vi "aggregator - i.vi"(5 "requested averaging interval":i32=1, 6 "first time":bool=TRUE, 7 "requested size":i32=1, 11 "number":cdb) -> (0 "interpolated average":cdb, 1 "mean array":cdb[](array[numeric]), 2 "interp array":cdb[](array[numeric]), 3 "Array":cdb[](array[numeric]), 4 "standard deviation":cdb[](array[numeric]))   [LabVIEW 2015]
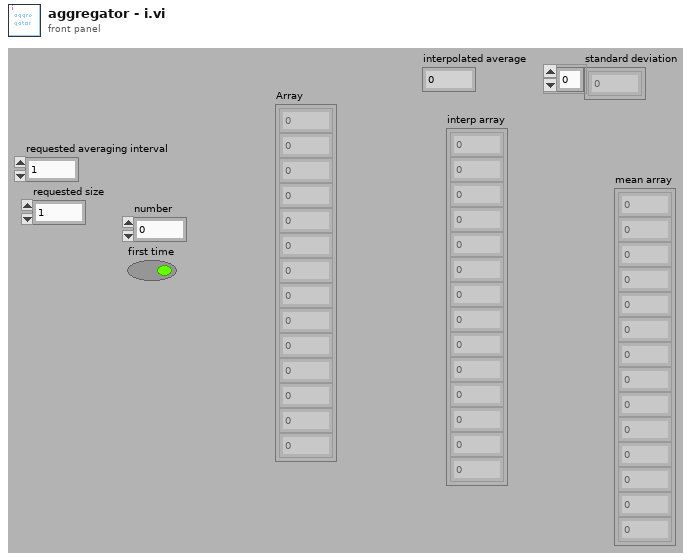
[diagram p1: front panel]
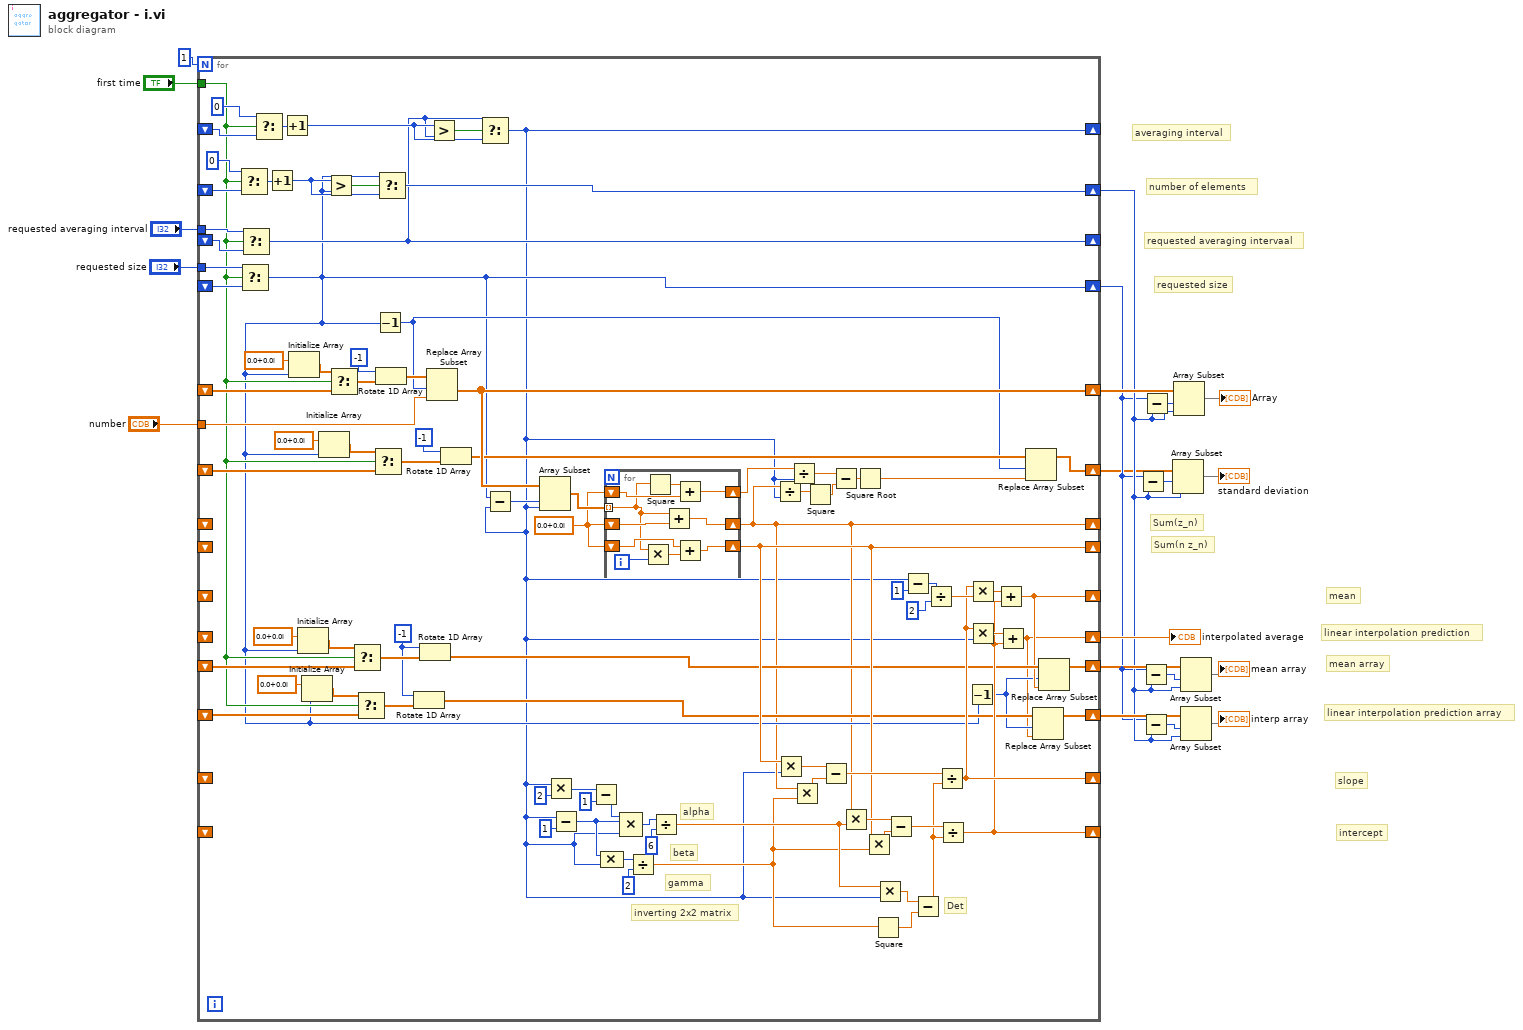
[diagram p0: block diagram]
diagram:
  # "averaging interval"
  # "requested averaging intervaal"
  # "linear interpolation prediction"
  # "mean"
  # "intercept"
  # "slope"
  # "linear interpolation prediction array"
  # "mean array"
  # "Sum(n z_n)"
  # "Sum(z_n)"
  # "requested size"
  # "number of elements"
  n1 = for {
    N: 1 -> [_]
    tunnel: "first time" -> [w31]
    shift-right: [w63] -> w3
    shift-left: _ -> [w110]
    tunnel: "requested size" -> [w100]
    tunnel: "number" -> [w104]
    shift-right: [w42] -> w16
    shift-left: _ -> [w106]
    shift-right: [w30] -> w2
    shift-left: _ -> [w99]
    shift-right: [w53] -> w10
    shift-left: _ -> [w94]
    shift-right: [w52] -> w7
    shift-left: _ -> [w93]
    shift-right: [w27] -> _
    shift-left: _ -> [_]
    shift-right: [w74] -> _
    shift-left: _ -> [_]
    shift-right: [w62] -> _
    shift-left: _ -> [_]
    shift-right: [w61] -> _
    shift-left: _ -> [_]
    shift-right: [w58] -> _
    shift-left: _ -> [_]
    shift-right: [w43] -> w6
    shift-left: _ -> [_]
    shift-right: [w26] -> _
    shift-left: _ -> [w47]
    shift-right: [w44] -> _
    shift-left: _ -> [w45]
    tunnel: "requested averaging interval" -> [w46]
    shift-right: [w33] -> w1
    shift-left: _ -> [w32]
    w55 = -1 ("n")
    w29 = cdb 0.0+0.0i
    # "inverting 2x2 matrix"
    # "Det"
    # "beta"
    # "gamma"
    # "alpha"
    n2 = Select(t=0, s=w31, f=w110) -> (s? t:f=w108:i32)
    n3 = Select(t=w100, s=w31, f=w99) -> (s? t:f=w30:i32)
    n4 = Select(t=w46, s=w31, f=w45) -> (s? t:f=w44:i32)
    n5 = Select(t=0, s=w31, f=w47) -> (s? t:f=w49:i32)
    n6 = Increment(x=w108) -> (x+1=w107:i32)
    n7 = Increment(x=w49) -> (x+1=w48:i32)
    n8 = Initialize Array(cdb 0.0+0.0i, w30) -> (w101:cdb[])
    n9 = Initialize Array(cdb 0.0+0.0i, w30) -> (w97:cdb[])
    n10 = Initialize Array(cdb 0.0+0.0i, w30) -> (w95:cdb[])
    n11 = Initialize Array(cdb 0.0+0.0i, w30) -> (w38:cdb[])
    n12 = Greater?(x=w107, y=w30) -> (0:w109:bool)
    n13 = Select(t=w101, s=w31, f=w106) -> (s? t:f=w92:cdb[])
    n14 = Select(t=w97, s=w31, f=w94) -> (s? t:f=w59:cdb[])
    n15 = Select(t=w95, s=w31, f=w93) -> (s? t:f=w56:cdb[])
    n16 = Select(t=w38, s=w31, f=w32) -> (s? t:f=w37:cdb[])
    n17 = Decrement(x=w30) -> (x-1=w34:i32)
    n18 = Rotate 1D Array(1:w92, 2:-1 ("n")) -> (0:w103:cdb[])
    n19 = Select(t=w30, s=w109, f=w107) -> (s? t:f=w63:i32)
    n20 = Rotate 1D Array(1:w56, 2:w55) -> (0:w57:cdb[])
    n21 = Rotate 1D Array(1:w59, 2:w55) -> (0:w60:cdb[])
    n22 = Replace Array Subset(array=w103, new element=w104, index=w34) -> (w42:cdb[])
    n23 = Greater?(x=w48, y=w44) -> (0:w50:bool)
    n24 = Rotate 1D Array(1:w37, 2:-1 ("n")) -> (0:w35:cdb[])
    n25 = Select(t=w44, s=w50, f=w48) -> (s? t:f=w26:i32)
    n26 = Subtract(x=w30, y=w26) -> (x-y=w41:i32)
    n27 = Array Subset(array=w42, index=w41, length=w26) -> (w40:cdb[])
    n28 = Multiply(x=w26, y=2 ("n")) -> (x*y=w88:i32)
    n29 = Subtract(x=w26, y=1 ("n")) -> (x-y=w84:i32)
    n30 = Subtract(x=w88, y=1 ("n")) -> (x-y=w87:i32)
    n31 = Compound Arithmetic op=MULTIPLY(w84, w26) -> (w82:i32)
    n32 = for {
      tunnel: w40 -> [w113] mode=indexing
      shift-right: [w121] -> w27
      shift-left: w29 -> [w120]
      shift-right: [w118] -> w74
      shift-left: w29 -> [w116]
      shift-right: [w115] -> w28
      shift-left: w29 -> [w114]
      i -> [w117]
      n33 = Multiply(x=w113, y=w117) -> (x*y=w119:cdb)
      n34 = Square(x=w113) -> (x^2=w112:cdb)
      n35 = Add(x=w113, y=w120) -> (x+y=w121:cdb)
      n36 = Add(x=w112, y=w114) -> (x+y=w115:cdb)
      n37 = Add(x=w116, y=w119) -> (x+y=w118:cdb)
    }
    n38 = Compound Arithmetic op=MULTIPLY(w87, w84, w26) -> (w86:i32)
    n39 = Divide(x=w82, y=2 ("n")) -> (x/y=w72:dbl)
    n40 = Divide(x=w86, y=6 ("n")) -> (x/y=w73:dbl)
    n41 = Divide(x=w27, y=w26) -> (x/y=w25:cdb)
    n42 = Multiply(x=w74, y=w26) -> (x*y=w78:cdb)
    n43 = Divide(x=w28, y=w26) -> (x/y=w24:cdb)
    n44 = Multiply(x=w27, y=w72) -> (x*y=w79:cdb)
    n45 = Square(x=w25) -> (x^2=w23:cdb)
    n46 = Subtract(x=w78, y=w79) -> (x-y=w77:cdb)
    n47 = Subtract(x=w24, y=w23) -> (x-y=w22:cdb)
    n48 = Multiply(x=w27, y=w73) -> (x*y=w75:cdb)
    n49 = Square Root(x=w22) -> (sqrt(x)=w21:cdb)
    n50 = Multiply(x=w74, y=w72) -> (x*y=w76:cdb)
    n51 = Square(x=w72) -> (x^2=w80:dbl)
    n52 = Multiply(x=w73, y=w26) -> (x*y=w81:dbl)
    n53 = Subtract(x=w75, y=w76) -> (x-y=w71:cdb)
    n54 = Subtract(x=w26, y=1 ("n")) -> (x-y=w68:i32)
    n55 = Subtract(x=w81, y=w80) -> (x-y=w70:dbl)
    n56 = Divide(x=w68, y=2 ("n")) -> (x/y=w66:dbl)
    n57 = Divide(x=w77, y=w70) -> (x/y=w62:cdb)
    n58 = Divide(x=w71, y=w70) -> (x/y=w61:cdb)
    n59 = Decrement(x=w30) -> (x-1=w54:i32)
    n60 = Multiply(x=w62, y=w66) -> (x*y=w65:cdb)
    n61 = Multiply(x=w62, y=w26) -> (x*y=w64:cdb)
    n62 = Add(x=w65, y=w61) -> (x+y=w58:cdb)
    n63 = Add(x=w64, y=w61) -> (x+y=w43:cdb)
    n64 = Replace Array Subset(array=w35, new element=w21, index=w34) -> (w33:cdb[])
    n65 = Replace Array Subset(array=w57, new element=w43, index=w54) -> (w52:cdb[])
    n66 = Replace Array Subset(array=w60, new element=w58, index=w54) -> (w53:cdb[])
  }
  "interpolated average" <- w6
  n67 = Subtract(x=w2, y=w3) -> (x-y=w5:i32)
  n68 = Subtract(x=w2, y=w3) -> (x-y=w11:i32)
  n69 = Subtract(x=w2, y=w3) -> (x-y=w8:i32)
  n70 = Subtract(x=w2, y=w3) -> (x-y=w14:i32)
  n71 = Array Subset(array=w1, index=w5, length=w3) -> (→"standard deviation":cdb[])
  n72 = Array Subset(array=w16, index=w14, length=w3) -> (→"Array":cdb[])
  n73 = Array Subset(array=w10, index=w11, length=w3) -> (→"mean array":cdb[])
  n74 = Array Subset(array=w7, index=w8, length=w3) -> (→"interp array":cdb[])
